vi "ReadAllHelper.vi"(0 "object in":refnum<class "MTEC_Async.lvclass">, 5 "error in (no error)":errorcluster) -> (14 "object out":refnum<class "MTEC_Async.lvclass">, 16 "DataOut":T3 {"meTEC_CH2_Temperature Stability" items=["Temperature regulation is not active", "Is not stable", "Is stable"]; "meTEC_CH1_Device Status" items=["Initializing", "Ready", "Run", "Error", "Bootloader", "Reset in Progress"]; "meTEC_CH1_Temperature Stability" items=["Temperature regulation is not active", "Is not stable", "Is stable"]}, 19 "error out":errorcluster)   [LabVIEW 2019, in "MTEC_Async.lvclass"]
uses:
  MTEC_Async.lvclass
  TEC LabVIEW Control Software v0.14/Source/LV Source/[meerstetter engineering TE Cooling]/TypeDefs/meTEC_ID 104_Device Status.ctl
  TEC LabVIEW Control Software v0.14/Source/LV Source/[meerstetter engineering TE Cooling]/TypeDefs/meTEC_ID 1200_Temperature is Stable.ctl
  MTEC_Async.lvclass/MTEC_Async.ctl
panel:
  out "meTEC_CH2_Sink Temperature [°C]":dbl caption="Sink Temperature [°C]" format="%.3f"
  out "meTEC_CH2_Object Temperature [°C]":dbl caption="Object Temperature [°C]" format="%.3f"
  out "meTEC_CH2_Act. Output Voltage [V]":dbl caption="Act. Output Voltage [V]" format="%.3f"
  out "meTEC_CH2_Act. Output Current [A]":dbl caption="Act. Output Current [A]" format="%.3f"
  out "meTEC_CH2_Temperature Stability":T1=1 caption="Temperature Stabilty" items=["Temperature regulation is not active", "Is not stable", "Is stable"]
  out "meTEC_CH1_Sink Temperature [°C]":dbl caption="Sink Temperature [°C]" format="%.3f"
  out "meTEC_CH1_Object Temperature [°C]":dbl caption="Object Temperature [°C]" format="%.3f"
  out "meTEC_CH1_Act. Output Voltage [V]":dbl caption="Act. Output Voltage [V]" format="%.3f"
  out "meTEC_CH1_Act. Output Current [A]":dbl caption="Act. Output Current [A]" format="%.3f"
  out "meTEC_CH1_Temperature Stability":T1=1 caption="Temperature Stabilty" items=["Temperature regulation is not active", "Is not stable", "Is stable"]
  out "meTEC_CH1_Device Status":T2=1 caption="Device Status" items=["Initializing", "Ready", "Run", "Error", "Bootloader", "Reset in Progress"]
  out "meTEC_CH1_Error No.":i32 caption="Error No."
  out "meTEC_CH1_Error Instance":i32 caption="Error Instance"
  out "meTEC_CH1_Error Parameter":i32 caption="Error Parameter"
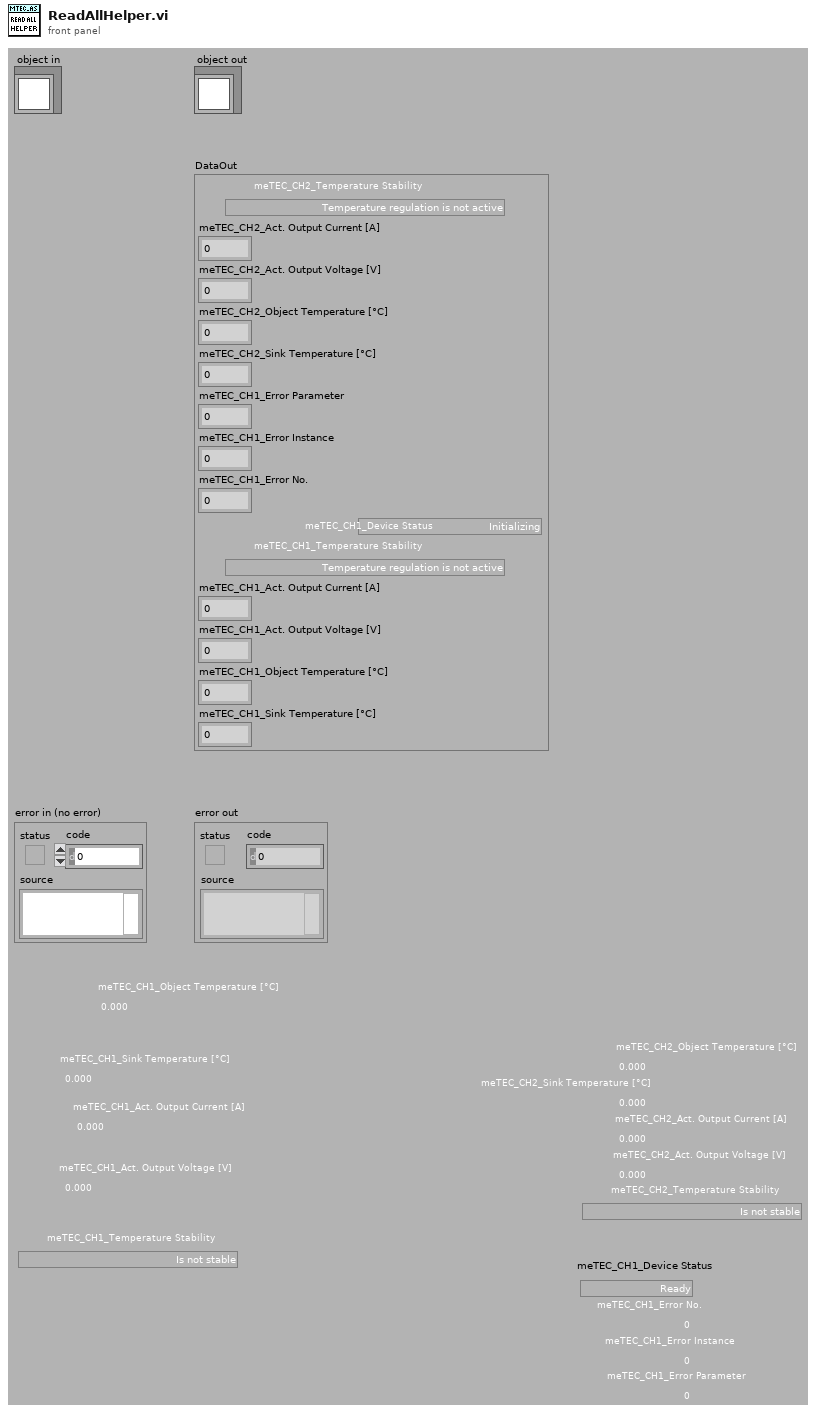
[diagram p1: front panel]
types:
  T1 = typedef "meTEC_ID 1200_Temperature is Stable.ctl" = i32
  T2 = typedef "meTEC_ID 104_Device Status.ctl" = i32
  T3 = cluster{"meTEC_CH2_Temperature Stability":T1, "meTEC_CH2_Act. Output Current [A]":dbl, "meTEC_CH2_Act. Output Voltage [V]":dbl, "meTEC_CH2_Object Temperature [°C]":dbl, "meTEC_CH2_Sink Temperature [°C]":dbl, "meTEC_CH1_Error Parameter":i32, "meTEC_CH1_Error Instance":i32, "meTEC_CH1_Error No.":i32, "meTEC_CH1_Device Status":T2, "meTEC_CH1_Temperature Stability":T1, "meTEC_CH1_Act. Output Current [A]":dbl, "meTEC_CH1_Act. Output Voltage [V]":dbl, "meTEC_CH1_Object Temperature [°C]":dbl, "meTEC_CH1_Sink Temperature [°C]":dbl}
  T4 = typedef "FGV_TE Controller.ctl" = cluster{"SVs":cluster{"Unused":dbl}, "PVs":cluster{"FW & HW Versions":cluster{"Device Type [I32]":i32, "Device Type [String]":string, "Firmware Version [I32]":i32, "Firmware Version [String]":string, "Hardware Version [I32]":i32, "Hardware Version [String]":string, "Serial No.":i32}, "TEC Configuration":T5, "Object Target Temperature Source_CH1":u8, "Object Target Temperature Source_CH2":u8}, "Front Panel References":T6}
  T5 = typedef "meTEC_Configuration.ctl" = cluster{"VISA resource name":refnum<visa-resource-name>, "Device Address":u16}
  T6 = typedef "FGV_Front Panel References.ctl" = cluster{"Main Loop Queue":refnum<queue>, "meTEC_Device Type":refnum<vi>, "meTEC_Serial No.":refnum<vi>, "meTEC_Hardware Version":refnum<vi>, "meTEC_Firmware Version":refnum<vi>, "meTEC_CH1_Object Target Temperature (ID 3000 / 50012) [°C]":refnum<vi>, "meTEC_CH1_Live Set Current (ID 50001) [A]":refnum<vi>, "meTEC_CH1_Live Set Voltage (ID 50002) [V]":refnum<vi>, "meTEC_CH1_Live Enable (ID 50000)":refnum<vi>, "meTEC_CH1_Input Selection (ID 2000)":refnum<vi>, "meTEC_CH1_Object Target Temp. Source Sel. (ID 50011)":refnum<vi>, "meTEC_CH2_Object Target Temperature (ID 3000 / 50012) [°C]":refnum<vi>, "meTEC_CH2_Live Set Current (ID 50001) [A]":refnum<vi>, "meTEC_CH2_Live Set Voltage (ID 50002) [V]":refnum<vi>, "meTEC_CH2_Live Enable (ID 50000)":refnum<vi>, "meTEC_CH2_Input Selection (ID 2000)":refnum<vi>, "meTEC_CH2_Object Target Temp. Source Sel. (ID 50011)":refnum<vi>, "meTEC_CH2_Object Temperature [°C]":refnum<vi>, "meTEC_CH2_Sink Temperature [°C]":refnum<vi>, "meTEC_CH2_Act. Output Current [A]":refnum<vi>, "meTEC_CH2_Act. Output Voltage [V]":refnum<vi>, "meTEC_CH2_Temperature Stability":refnum<vi>, "Monitor Chart_CH2":refnum<vi>, "meTEC_Initialize Device":refnum<vi>}
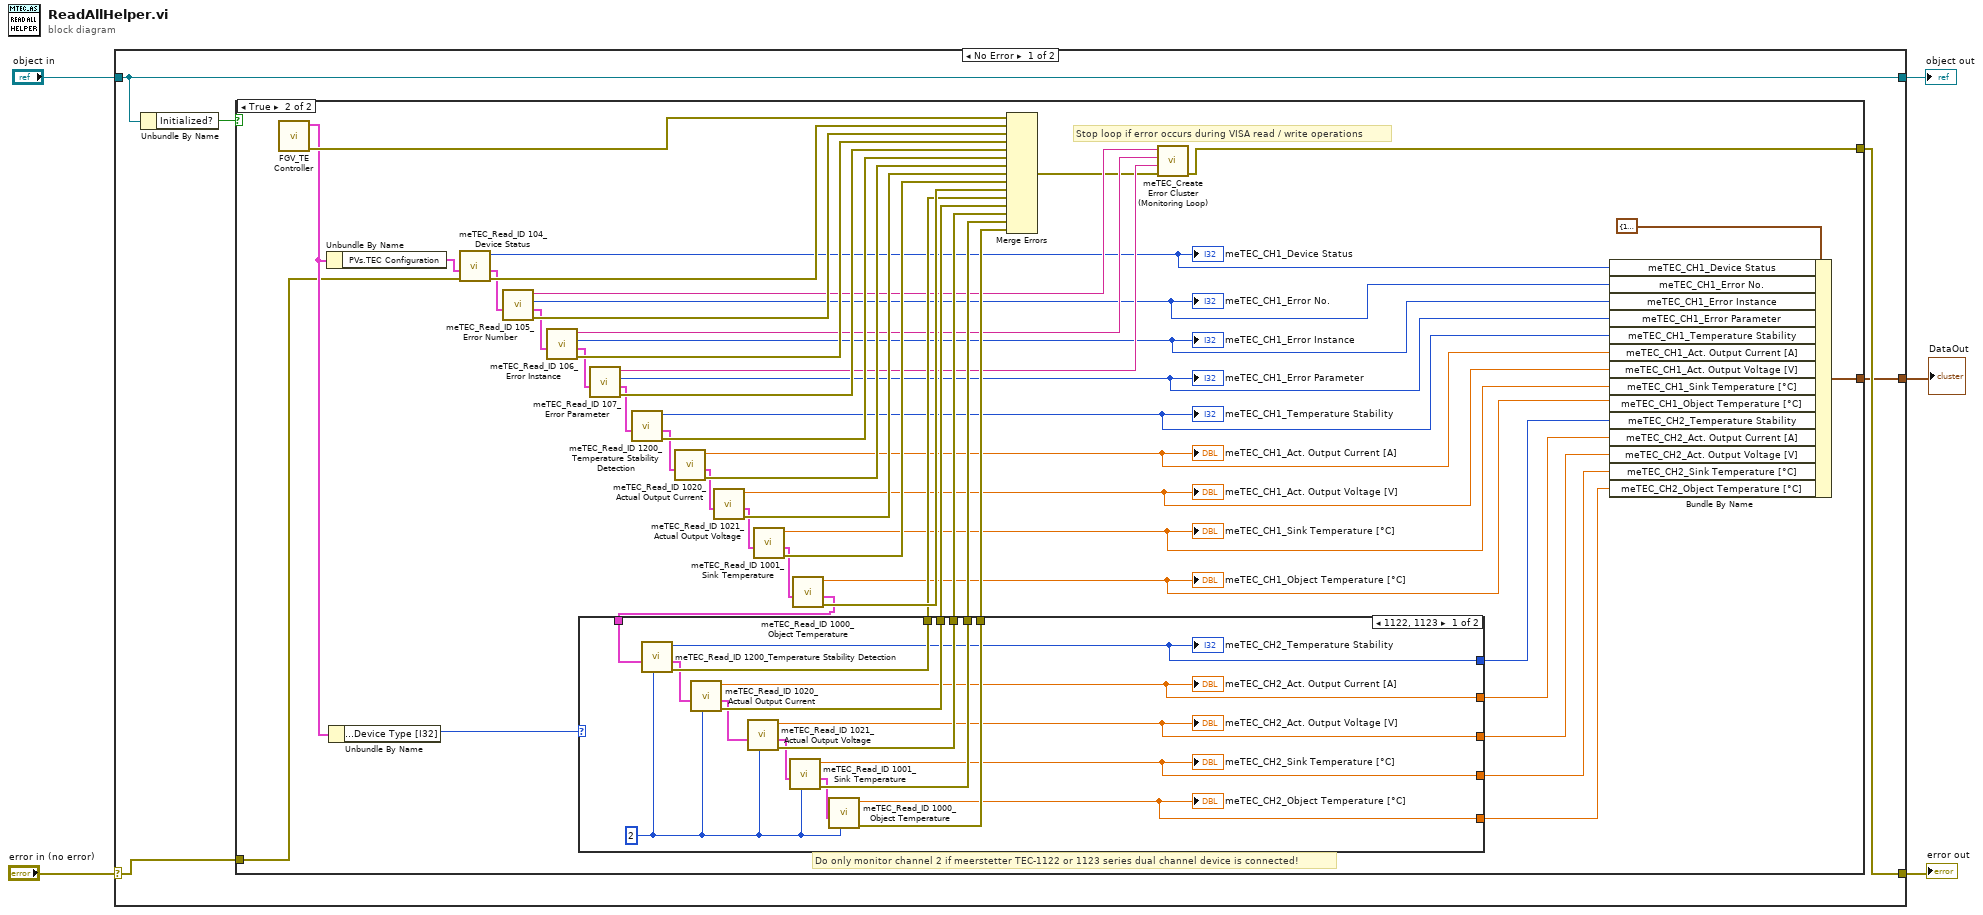
[diagram p0: block diagram]
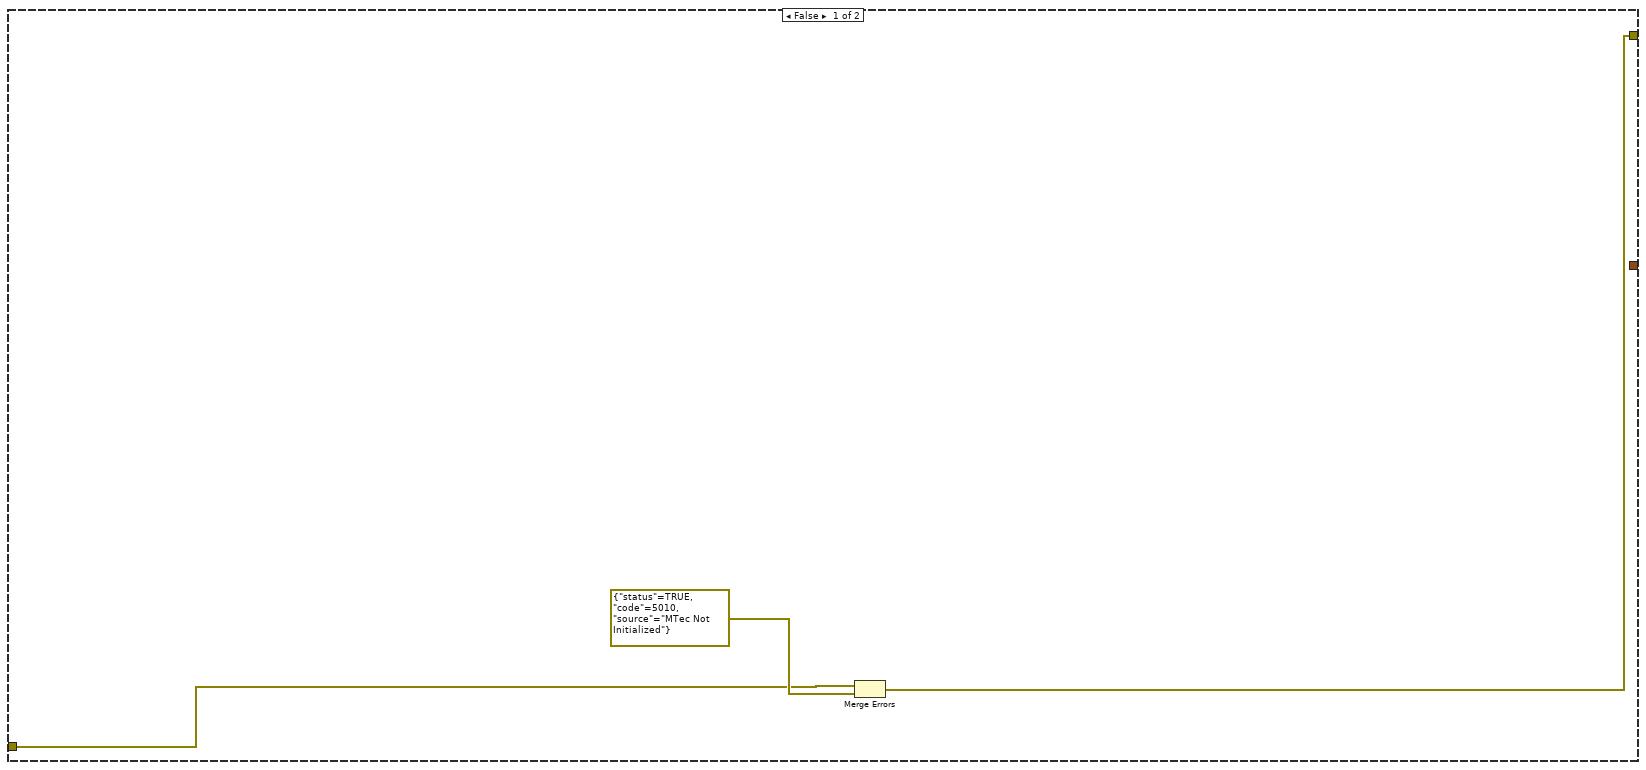
[diagram p2: hidden frame]
diagram:
  n1 = case shown="No Error" "error in (no error)" {
    selector: "error in (no error)" -> [w8 w80]
    tunnel: [w7 w80] -> w4
    tunnel: [w9 w79] -> w2
    tunnel: "object in" -> [w9 w79]
    tunnel: [w6 _] -> w1
    frame No Error {
      n2 = Unbundle By Name(w9) -> ("Initialized?"=w10:bool)
      n3 = case shown="True" w10 {
        tunnel: w8 -> [w12 w25]
        tunnel: [w11 w24] -> w7
        tunnel: [_ w23] -> w6
        frame False {
          n4 = Merge Errors(w12, errorcluster {"status"=TRUE, "code"=5010, "source"="MTec Not Initialized"} ("error in (no error)")) -> (w11:errorcluster)
        }
        frame True {
          # "Do only monitor channel 2 if meerstetter TEC-1122 or 1123 series dual channel device is connected!"
          # "Stop loop if error occurs during VISA read / write operations"
          n5 = call "FGV_TE Controller.vi"() -> ("error out"=w62:errorcluster, "FGV_TEC_OUT"=w47:T4)  [unwired: 10 in]
          n6 = Unbundle By Name(w47) -> ("PVs.TEC Configuration"=w45:T5)
          n7 = Unbundle By Name(w47) -> ("PVs.FW & HW Versions.Device Type [I32]"=w46:i32)
          n8 = call "meTEC_Read_ID 104_Device Status.vi"("error in (no error)"=w25, "TEC Configuration_IN"=w45) -> ("error out"=w56:errorcluster, "TEC Configuration_OUT"=w22:T5, "Device Status (ID 104) [I32]"=w39:i32)  [unwired: 7 in]
          "meTEC_CH1_Device Status" <- w39
          n9 = call "meTEC_Read_ID 105_Error Number.vi"("TEC Configuration_IN"=w22) -> ("error out"=w55:errorcluster, "TEC Configuration_OUT"=w21:T5, "Error Number (ID 105) [I32]"=w38:i32, "Error Number (ID 105) [String]"=w42:string)  [unwired: 7 in]
          "meTEC_CH1_Error No." <- w38
          n10 = call "meTEC_Read_ID 106_Error Instance.vi"("TEC Configuration_IN"=w21) -> ("error out"=w54:errorcluster, "TEC Configuration_OUT"=w20:T5, "Error Instance (ID 106) [I32]"=w37:i32, "Error Instance (ID 106) [String]"=w43:string)  [unwired: 7 in]
          "meTEC_CH1_Error Instance" <- w37
          n11 = call "meTEC_Read_ID 107_Error Parameter.vi"("TEC Configuration_IN"=w20) -> ("error out"=w53:errorcluster, "TEC Configuration_OUT"=w19:T5, "Error Parameter (ID 107) [I32]"=w36:i32, "Error Parameter (ID 107) [String]"=w44:string)  [unwired: 7 in]
          "meTEC_CH1_Error Parameter" <- w36
          n12 = call "meTEC_Read_ID 1200_Temperature Stability Detection.vi"("TEC Configuration_IN"=w19) -> ("error out"=w61:errorcluster, "TEC Configuration_OUT"=w18:T5, "Temperature is Stable? [I32)] (ID 1200)"=w35:i32)  [unwired: 7 in, 1 out]
          "meTEC_CH1_Temperature Stability" <- w35
          n13 = call "meTEC_Read_ID 1020_Actual Output Current.vi"("TEC Configuration_IN"=w18) -> ("error out"=w60:errorcluster, "TEC Configuration_OUT"=w17:T5, "Act. Output Current [A] (ID 1020)"=w34:dbl)  [unwired: 8 in]
          "meTEC_CH1_Act. Output Current [A]" <- w34
          n14 = call "meTEC_Read_ID 1021_Actual Output Voltage.vi"("TEC Configuration_IN"=w17) -> ("error out"=w59:errorcluster, "TEC Configuration_OUT"=w16:T5, "Act. Output Voltage [A] (ID 1021)"=w33:dbl)  [unwired: 8 in]
          "meTEC_CH1_Act. Output Voltage [V]" <- w33
          n15 = call "meTEC_Read_ID 1001_Sink Temperature.vi"("TEC Configuration_IN"=w16) -> ("error out"=w58:errorcluster, "TEC Configuration_OUT"=w15:T5, "Sink Temperature [°C] (ID 1001)"=w32:dbl)  [unwired: 8 in]
          "meTEC_CH1_Sink Temperature [°C]" <- w32
          n16 = call "meTEC_Read_ID 1000_Object Temperature.vi"("TEC Configuration_IN"=w15) -> ("error out"=w57:errorcluster, "TEC Configuration_OUT"=w14:T5, "Object Temperature [°C] (ID 1000)"=w31:dbl)  [unwired: 8 in]
          "meTEC_CH1_Object Temperature [°C]" <- w31
          n17 = case shown="1122, 1123" w46 {
            tunnel: w14 -> [w78 _]
            tunnel: [w77 _] -> w52
            tunnel: [w76 _] -> w51
            tunnel: [w75 _] -> w50
            tunnel: [w74 _] -> w49
            tunnel: [w73 _] -> w48
            tunnel: [w71 _] -> w30
            tunnel: [w70 _] -> w29
            tunnel: [w69 _] -> w28
            tunnel: [w68 _] -> w27
            tunnel: [w67 _] -> w26
            frame 1122, 1123 {
              w72 = u8 2 ("Instance (1)")
              n18 = call "meTEC_Read_ID 1200_Temperature Stability Detection.vi"("Instance (1)"=w72, "TEC Configuration_IN"=w78) -> ("error out"=w77:errorcluster, "TEC Configuration_OUT"=w66:T5, "Temperature is Stable? [I32)] (ID 1200)"=w71:i32)  [unwired: 6 in, 1 out]
              "meTEC_CH2_Temperature Stability" <- w71
              n19 = call "meTEC_Read_ID 1020_Actual Output Current.vi"("Instance (1)"=w72, "TEC Configuration_IN"=w66) -> ("error out"=w76:errorcluster, "TEC Configuration_OUT"=w65:T5, "Act. Output Current [A] (ID 1020)"=w70:dbl)  [unwired: 7 in]
              "meTEC_CH2_Act. Output Current [A]" <- w70
              n20 = call "meTEC_Read_ID 1021_Actual Output Voltage.vi"("Instance (1)"=w72, "TEC Configuration_IN"=w65) -> ("error out"=w75:errorcluster, "TEC Configuration_OUT"=w64:T5, "Act. Output Voltage [A] (ID 1021)"=w69:dbl)  [unwired: 7 in]
              "meTEC_CH2_Act. Output Voltage [V]" <- w69
              n21 = call "meTEC_Read_ID 1001_Sink Temperature.vi"("Instance (1)"=w72, "TEC Configuration_IN"=w64) -> ("error out"=w74:errorcluster, "TEC Configuration_OUT"=w63:T5, "Sink Temperature [°C] (ID 1001)"=w68:dbl)  [unwired: 7 in]
              "meTEC_CH2_Sink Temperature [°C]" <- w68
              n22 = call "meTEC_Read_ID 1000_Object Temperature.vi"("Instance (1)"=w72, "TEC Configuration_IN"=w63) -> ("error out"=w73:errorcluster, "Object Temperature [°C] (ID 1000)"=w67:dbl)  [unwired: 7 in, 1 out]
              "meTEC_CH2_Object Temperature [°C]" <- w67
            }
            frame 1089..1091, Default {
            }
          }
          n23 = Merge Errors(w62, w56, w55, w54, w53, w61, w60, w59, w58, w57, w52, w51, w50, w49, w48) -> (w41:errorcluster)
          n24 = call "meTEC_Create Error Cluster (Monitoring Loop).vi"("error in (no error)"=w41, "Error Parameter"=w44, "Error Instance"=w43, "Error Number"=w42) -> ("error out"=w24:errorcluster)  [unwired: 7 in]
          n25 = Bundle By Name(cluster=T3 {"meTEC_CH2_Temperature Stability"=1, "meTEC_CH2_Act. Output Current [A]"=0.0, "meTEC_CH2_Act. Output Voltage [V]"=0.0, "meTEC_CH2_Object Temperature [°C]"=0.0, "meTEC_CH2_Sink Temperature [°C]"=0.0, "meTEC_CH1_Error Parameter"=0, "meTEC_CH1_Error Instance"=0, "meTEC_CH1_Error No."=0, "meTEC_CH1_Device Status"=1, "meTEC_CH1_Temperature Stability"=1, "meTEC_CH1_Act. Output Current [A]"=0.0, "meTEC_CH1_Act. Output Voltage [V]"=0.0, "meTEC_CH1_Object Temperature [°C]"=0.0, "meTEC_CH1_Sink Temperature [°C]"=0.0} ("Cluster"), "meTEC_CH1_Device Status"=w39, "meTEC_CH1_Error No."=w38, "meTEC_CH1_Error Instance"=w37, "meTEC_CH1_Error Parameter"=w36, "meTEC_CH1_Temperature Stability"=w35, "meTEC_CH1_Act. Output Current [A]"=w34, "meTEC_CH1_Act. Output Voltage [V]"=w33, "meTEC_CH1_Sink Temperature [°C]"=w32, "meTEC_CH1_Object Temperature [°C]"=w31, "meTEC_CH2_Temperature Stability"=w30, "meTEC_CH2_Act. Output Current [A]"=w29, "meTEC_CH2_Act. Output Voltage [V]"=w28, "meTEC_CH2_Sink Temperature [°C]"=w27, "meTEC_CH2_Object Temperature [°C]"=w26) -> (w23:T3)
        }
      }
    }
    frame Error {
    }
  }
  "error out" <- w4
  "object out" <- w2
  "DataOut" <- w1
